vi "Nocluster.vi"(11 "Array In":refnum<vi>[](array[refnum])) -> (2 "NoCluster":bool, 3 "Array Out":refnum<vi>[](array[refnum]))   [LabVIEW 2015]
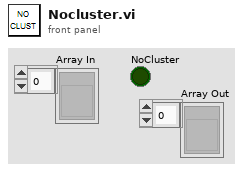
[diagram p1: front panel]
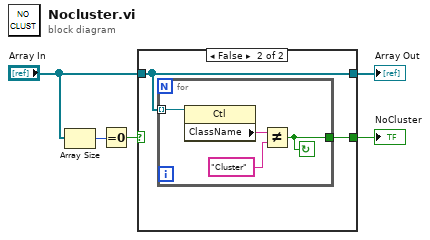
[diagram p0: block diagram]
diagram:
  n1 = Array Size(array="Array In") -> (size(s)=w3:i32)
  n2 = Equal To 0?(x=w3) -> (x = 0?=w2:bool)
  n3 = case shown="False" w2 {
    selector: w2 -> [w7 _]
    tunnel: [w7 w9] -> w5
    tunnel: "Array In" -> [w6 w8]
    tunnel: [w6 w8] -> w1
    frame True {
    }
    frame False {
      n4 = for {
        tunnel: w8 -> [w13] mode=indexing
        tunnel: [w10] -> w9
        stop <- w10 continue-if-true
        n5 = property class="Ctl"(reference=w13) -> ("ClassName"=w12:string)  [unwired: 1 in, 2 out]
        n6 = Not Equal?(x=w12, y="Cluster") -> (x != y?=w10:bool)
      }
    }
  }
  "NoCluster" <- w5
  "Array Out" <- w1
